vi "Simple Spectrometer Demo.vi"() -> ()   [LabVIEW 2013]
uses:
  C:/GEECS/Developers Version/source/Device Driver/Qred/Library/RgbDriverKit/Sample code/LabView/RgbDriverKit.dll
  RgbDriverKit.dll
  <vilib>/Utility/file.llb/Write To Spreadsheet File (DBL).vi
panel:
  in  "timeout (ms)":u32=1000
  out "Timed out":bool
  in  "UseExternalTrigger":bool
  in  "start path":path=path "N:/data/Y2018/05-May/18_0529/qred tests"
  out "error out 2":errorcluster
  out "Device":string
  out "Measured spectrum":cluster{"Y":dbl[], "Y":dbl[]}[](graph)
  out "error out":errorcluster
  in  "error in (no error)":errorcluster
  out "Status":i32(ring) items=["Idle"=0, "WaitingForTrigger"=1, "TakingSpectrum"=2, "HasData"=3, "Error"=-3, "Busy"=-2, "NotReady"=-1]
  in  "Use sensitivity calibration":bool
  in  "Exposure time [sec]":dbl=0.1 format="%#_6f"
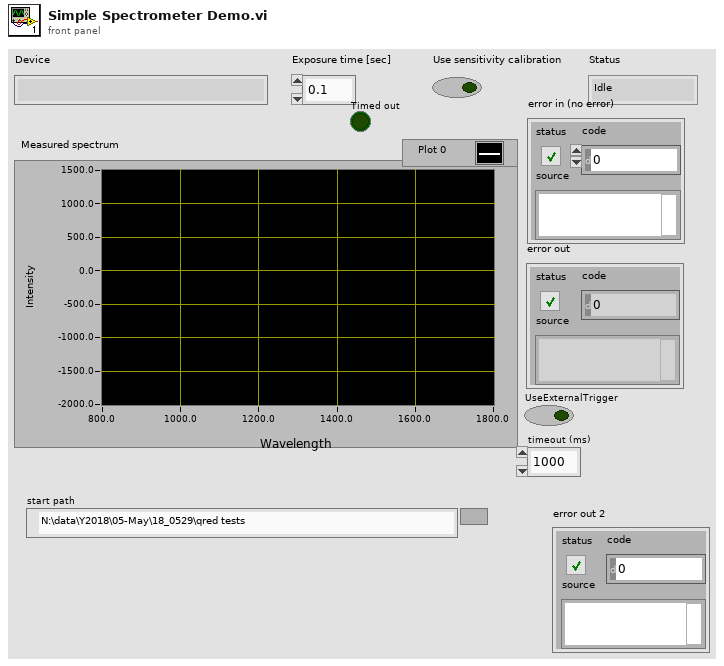
[diagram p1: front panel]
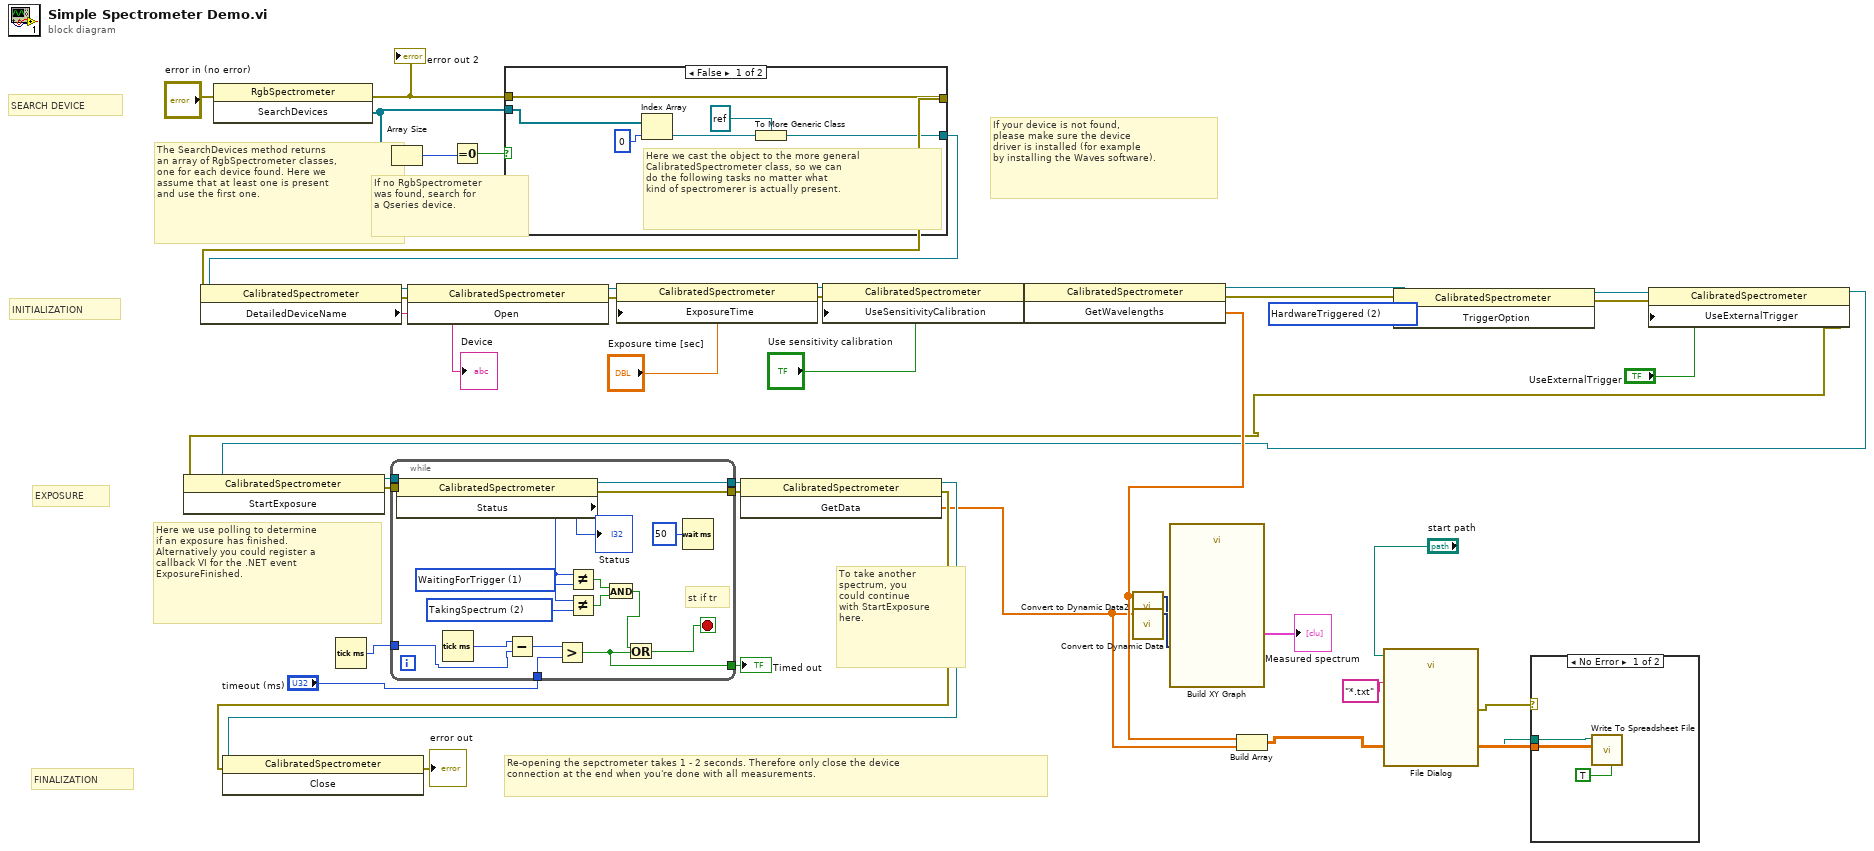
[diagram p0: block diagram]
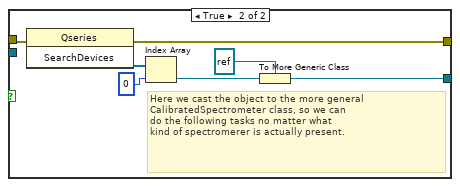
[diagram p3: hidden frame]
diagram:
  w12 = 2 items=["FreeRunningTriggerEnd", "FreeRunningTriggerStart", "HardwareTriggered"] ("TriggerOption")
  # "SEARCH DEVICE"
  # "If no RgbSpectrometer\nwas found, search for\na Qseries device."
  # "Re-opening the sepctrometer takes 1 - 2 seconds. Therefore only close the device\nconnection at the end when you're done with all measurements."
  # "To take another\nspectrum, you\ncould continue\nwith StartExposure\nhere."
  # "If your device is not found,\nplease make sure the device\ndriver is installed (for example\nby installing the Waves software)."
  # "FINALIZATION"
  # "EXPOSURE"
  # "INITIALIZATION"
  # "Here we use polling to determine\nif an exposure has finished.\nAlternatively you could register a\ncallback VI for the .NET event\nExposureFinished."
  # "The SearchDevices method returns\nan array of RgbSpectrometer classes,\none for each device found. Here we\nassume that at least one is present\nand use the first one."
  n1 = invoke class="RgbSpectrometer" method="SearchDevices"(error in="error in (no error)") -> (error out=w25:errorcluster, "SearchDevices"=w24:refnum<k24>[])  [unwired: 2 in, 1 out]
  "error out 2" <- w25
  n2 = Tick Count (ms)() -> (millisecond timer value=w3:u32)
  n3 = Array Size(array=w24) -> (size(s)=w22:i32)
  n4 = Equal To 0?(x=w22) -> (x = 0?=w23:bool)
  n5 = case shown="False" w23 {
    tunnel: w25 -> [w49 w59]
    tunnel: w24 -> [w48 _]
    tunnel: [w47 w53] -> w20
    tunnel: [w49 w56] -> w21
    frame False {
      # "Here we cast the object to the more general\nCalibratedSpectrometer class, so we can\ndo the following tasks no matter what\nkind of spectromerer is actually present."
      n6 = Index Array(array=w48, index=0) -> (element=w51:refnum<k24>)
      n7 = To More Generic Class(target class=refnum<k24> refnum, reference=w51) -> (generic class reference=w47:refnum<k24>)
    }
    frame True {
      # "Here we cast the object to the more general\nCalibratedSpectrometer class, so we can\ndo the following tasks no matter what\nkind of spectromerer is actually present."
      n8 = invoke class="Qseries" method="SearchDevices"(error in=w59) -> (error out=w56:errorcluster, "SearchDevices"=w58:refnum<k24>[])  [unwired: 2 in, 1 out]
      n9 = Index Array(array=w58, index=0) -> (element=w55:refnum<k24>)
      n10 = To More Generic Class(target class=refnum<k24> refnum, reference=w55) -> (generic class reference=w53:refnum<k24>)
    }
  }
  n11 = property class="CalibratedSpectrometer"(reference=w20, error in=w21) -> (reference out=w28:refnum<k24>, error out=w27:errorcluster, "DetailedDeviceName"=→"Device":string)
  n12 = invoke class="CalibratedSpectrometer" method="Open"(reference=w28, error in=w27) -> (reference out=w45:refnum<k24>, error out=w46:errorcluster)  [unwired: 1 in, 1 out]
  n13 = property class="CalibratedSpectrometer"(reference=w45, error in=w46, "ExposureTime"="Exposure time [sec]") -> (reference out=w43:refnum<k24>, error out=w42:errorcluster)
  n14 = property class="CalibratedSpectrometer"(reference=w43, error in=w42, "UseSensitivityCalibration"="Use sensitivity calibration") -> (reference out=w31:refnum<k24>, error out=w30:errorcluster)
  n15 = invoke class="CalibratedSpectrometer" method="GetWavelengths"(reference=w31, error in=w30) -> (reference out=w10:refnum<k24>, error out=w9:errorcluster, "GetWavelengths"=w18:dbl[])  [unwired: 1 in]
  n16 = call "Convert to Dynamic Data2"("Array"=w18) -> ("Dynamic Data Type"=w29:dynamicdata)  [unwired: 3 in]
  n17 = call "File Dialog"("start path"="start path", "pattern (all files)"="*.txt" ("pattern label")) -> ("selected path"=w14:path, "error out"=w4:errorcluster)  [unwired: 10 in, 2 out]
  n18 = property class="CalibratedSpectrometer"(reference=w10, error in=w9, "TriggerOption"=w12) -> (reference out=w8:refnum<k24>, error out=w7:errorcluster)
  n19 = property class="CalibratedSpectrometer"(reference=w8, error in=w7, "UseExternalTrigger"="UseExternalTrigger") -> (reference out=w6:refnum<k24>, error out=w5:errorcluster)
  n20 = invoke class="CalibratedSpectrometer" method="StartExposure"(reference=w6, error in=w5) -> (reference out=w40:refnum<k24>, error out=w39:errorcluster)  [unwired: 1 in, 1 out]
  n21 = while {
    tunnel: w40 -> [w75]
    tunnel: w39 -> [w74]
    tunnel: [w73] -> w38
    tunnel: [w72] -> w37
    tunnel: w3 -> [w64]
    tunnel: "timeout (ms)" -> [w62]
    tunnel: [w60] -> w1
    stop <- w61 stop-if-true
    w70 = 2 items=["Idle"=0, "WaitingForTrigger"=1, "TakingSpectrum"=2, "HasData"=3, "Error"=-3, "Busy"=-2, "NotReady"=-1] ("Status")
    w71 = 1 items=["Idle"=0, "WaitingForTrigger"=1, "TakingSpectrum"=2, "HasData"=3, "Error"=-3, "Busy"=-2, "NotReady"=-1] ("Status")
    # "st if tr"
    n22 = property class="CalibratedSpectrometer"(reference=w75, error in=w74) -> (reference out=w73:refnum<k24>, error out=w72:errorcluster, "Status"=w67:i32)
    "Status" <- w67
    n23 = Tick Count (ms)() -> (millisecond timer value=w65:u32)
    n24 = Subtract(x=w65, y=w64) -> (x-y=w63:u32)
    n25 = Greater?(x=w63, y=w62) -> (0:w60:bool)
    n26 = Not Equal?(x=w67, y=w71) -> (x != y?=w69:bool)
    n27 = Not Equal?(x=w67, y=w70) -> (x != y?=w68:bool)
    n28 = And(x=w69, y=w68) -> (x .and. y?=w66:bool)
    n29 = Or(x=w66, y=w60) -> (x .or. y?=w61:bool)
    n30 = Wait (ms)(milliseconds to wait=u32 50) -> ()  [unwired: 1 out]
  }
  "Timed out" <- w1
  n31 = invoke class="CalibratedSpectrometer" method="GetData"(reference=w38, error in=w37) -> (reference out=w35:refnum<k24>, error out=w36:errorcluster, "GetData"=w17:sgl[])  [unwired: 1 in]
  n32 = invoke class="CalibratedSpectrometer" method="Close"(reference=w35, error in=w36) -> (error out=→"error out":errorcluster)  [unwired: 1 in, 2 out]
  n33 = call "Convert to Dynamic Data"("Array"=w17) -> ("Dynamic Data Type"=w32:dynamicdata)  [unwired: 3 in]
  n34 = call "Build XY Graph"("Y Input"=w32, "X Input"=w29) -> ("XY Graph"=→"Measured spectrum":cluster{"Y":dbl[], "Y":dbl[]}[])  [unwired: 3 in, 6 out]
  n35 = Build Array(w18, w17) -> (w16:dbl[][])
  n36 = case shown="No Error" w4 {
    tunnel: w16 -> [w79 _]
    tunnel: w14 -> [w78 _]
    frame No Error {
      n37 = call-poly <vilib>:"Write To Spreadsheet File.vi"("transpose? (no:F)"=TRUE, "2D data"=w79, "file path (dialog if empty)"=w78) -> ()  [unwired: 5 in, 1 out]
    }
    frame Error {
    }
  }
